vi "dataInArrayAtIndex.vi"(0 "index":i32, 1 "Array":variant[](array[variant])) -> (2 "data":variant)   [LabVIEW 2015]
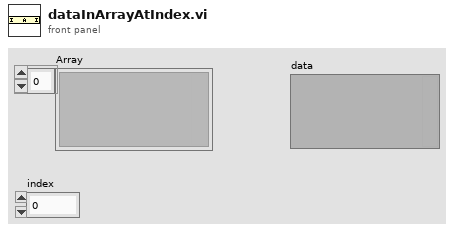
[diagram p1: front panel]
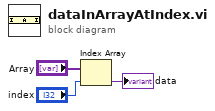
[diagram p0: block diagram]
diagram:
  n1 = Index Array(array="Array", index="index") -> (element=→"data":variant)
